vi "Long to Hexa.vi"(3 "Long":i32) -> (1 "Hexa":string)   [LabVIEW 2017]
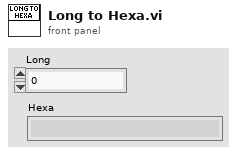
[diagram p1: front panel]
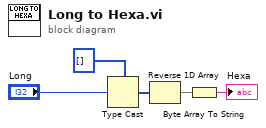
[diagram p0: block diagram]
diagram:
  n1 = Type Cast(type=u8[] [] ("typ"), x="Long") -> (*(type *) &x=w4:u8[])
  n2 = Reverse 1D Array(array=w4) -> (reversed array=w5:u8[])
  n3 = Byte Array To String(unsigned byte array=w5) -> (string=→"Hexa":string)
